vi "Integrator Trapez.vi"   [LabVIEW 2014]
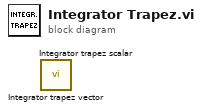
[diagram p0: block diagram]
diagram:
  n1 = call "Integrator trapez vector.vi"() -> ()  [unwired: 6 in, 1 out]
  n2 = call "Integrator trapez scalar.vi"() -> ()  [unwired: 6 in, 1 out]
